vi "exec.vi"(8 "error in (no error)":errorcluster, 11 "SelectGrating in":refnum<class "SelectGrating.lvclass">) -> (0 "error out":errorcluster, 3 "SelectGrating out":refnum<class "SelectGrating.lvclass">)   [LabVIEW 2020, in "SelectGrating.lvclass"]
uses:
  SelectGrating.lvclass
  C:/Users/Eric Coughlin/repos/ss_monochromator/WindowsController/Commands/Command/Command.lvclass
  Command/Command.lvclass/Command.ctl
  SelectGrating.lvclass/SelectGrating.ctl
  Command/Command.lvclass
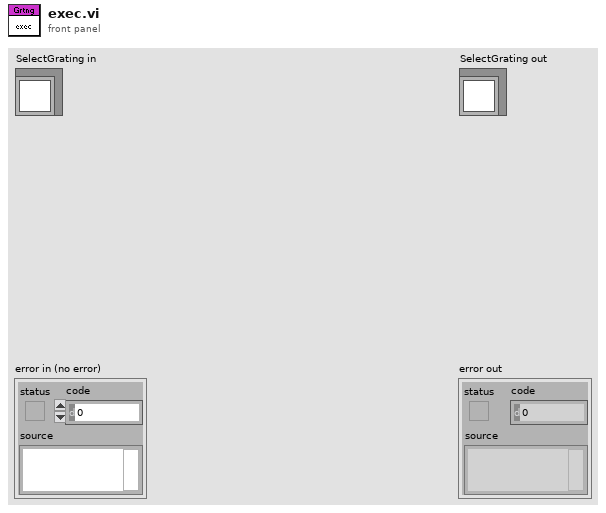
[diagram p1: front panel]
types:
  T1 = typedef "GratingType.ctl" = enum16{"Blue", "Red", "Mirror"}
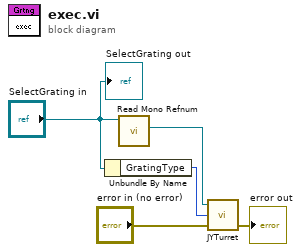
[diagram p0: block diagram]
diagram:
  n1 = Unbundle By Name("SelectGrating in") -> ("GratingType"=w4:T1)
  n2 = call "Read Mono Refnum.vi"("Command in"="SelectGrating in") -> ("Mono Refnum"=w3:refnum<k7>)  [unwired: 8 in, 2 out]
  n3 = call "JYTurret.vi"("error in (no error)"="error in (no error)", "Grating Index"=w4, "JYMONOLib.IJYMonoReqd"=w3) -> ("error out"=→"error out":errorcluster)  [unwired: 2 out]
  "SelectGrating out" <- "SelectGrating in"
